vi "Update Analysis DVR U16.vi"(8 "error in (no error)":errorcluster, 9 "images":refnum<data-value>[](array[refnum]), 10 "Analysis Image":dbl[][](array[numeric]), 11 "Analysis Graph in":refnum<class "Analysis Graph.lvclass">) -> (0 "error out":errorcluster, 1 "pixel signal roied":u16[](array[numeric]), 2 "Cursor.Cursor Position":T1, 3 "Analysis Graph out":refnum<class "Analysis Graph.lvclass">)   [LabVIEW 2023, in "Analysis Graph.lvclass"]
uses:
  Analysis Graph.lvclass
  Series Graph/Series Graph.lvclass
  Detail Graph/Detail Graph.lvclass
  <vilib>/Utility/miscctls.llb/LVPointDoubleTypeDef.ctl
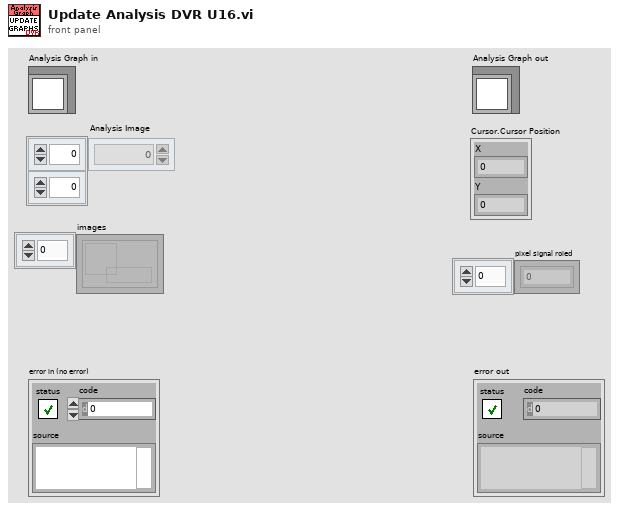
[diagram p1: front panel]
types:
  T1 = typedef "LVPointDoubleTypeDef.ctl" = cluster{"X":dbl, "Y":dbl}
  T2 = cluster{"ROI X":cluster{"Index":u32, "Length":u32}, "ROI Y":cluster{"Index":u32, "Length":u32}, "ROI Z":cluster{"Index":u32, "Length":u32}}
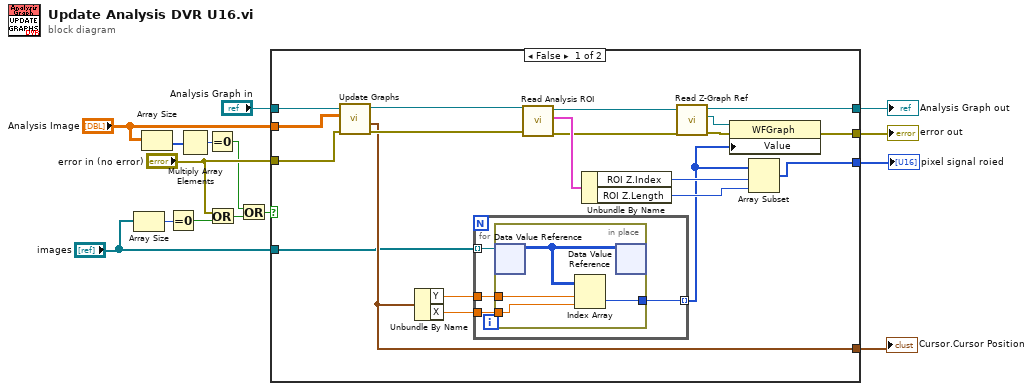
[diagram p0: block diagram]
diagram:
  n1 = Array Size(array="images") -> (size(s)=w8:i32)
  n2 = Array Size(array="Analysis Image") -> (size(s)=w4:i32[])
  n3 = Equal To 0?(x=w8) -> (x = 0?=w12:bool)
  n4 = Multiply Array Elements(1:w4) -> (0:w3:i32)
  n5 = Equal To 0?(x=w3) -> (x = 0?=w1:bool)
  n6 = Or(x="error in (no error)", y=w12) -> (x .or. y?=w11:bool)
  n7 = Or(x=w1, y=w11) -> (x .or. y?=w2:bool)
  n8 = case shown="False" w2 {
    tunnel: [w31 w44] -> w15
    tunnel: [w35 w45] -> w13
    tunnel: "Analysis Graph in" -> [w27 w45]
    tunnel: "error in (no error)" -> [w26 w44]
    tunnel: "Analysis Image" -> [w32 _]
    tunnel: "images" -> [w18 _]
    tunnel: [w19 _] -> w9
    tunnel: [w16 _] -> w6
    frame False {
      n9 = call "Update Graphs.vi"("error in (no error)"=w26, "image"=w32, "Detail Graph in"=w27) -> ("error out"=w29:errorcluster, "Cursor.Cursor Position"=w19:T1, "Detail Graph out"=w23:refnum<class "Analysis Graph.lvclass">)  [unwired: 6 in]
      n10 = Unbundle By Name(w19) -> ("Y"=w21:dbl, "X"=w20:dbl)
      n11 = for {
        tunnel: w18 -> [w39] mode=indexing
        tunnel: w21 -> [w38]
        tunnel: w20 -> [w37]
        tunnel: [w36] -> w17 mode=indexing
        n12 = in-place {
          in-place-border: w38 -> [w43]
          in-place-border: w37 -> [w42]
          in-place-border: [w41] -> w36
          n13 = in-place-dvr #1(w39) -> (w40:u16[][])  [unwired: 1 out]
          n14 = Index Array(array=w40, index (row)=w43, index (col)=w42) -> (element=w41:u16)
          n15 = in-place-dvr #1(w40) -> ()  [unwired: 2 out]
        }
      }
      n16 = call "Read Analysis ROI.vi"("error in (no error)"=w29, "Analysis Graph in"=w23) -> ("error out"=w28:errorcluster, "ROI XYZ"=w30:T2, "Analysis Graph out"=w22:refnum<class "Analysis Graph.lvclass">)  [unwired: 7 in]
      n17 = Unbundle By Name(w30) -> ("ROI Z.Index"=w25:u32, "ROI Z.Length"=w24:u32)
      n18 = call "Read Z-Graph Ref.vi"("error in (no error)"=w28, "Series Graph in"=w22) -> ("error out"=w33:errorcluster, "Z-Graph Ref"=w34:refnum<vi>, "Series Graph out"=w35:refnum<class "Analysis Graph.lvclass">)  [unwired: 7 in]
      n19 = property class="WFGraph"(reference=w34, error in=w33, "Value"=w17) -> (error out=w31:errorcluster)  [unwired: 1 out]
      n20 = Array Subset(array=w17, index=w25, length=w24) -> (w16:u16[])
    }
    frame True {
    }
  }
  "error out" <- w15
  "Analysis Graph out" <- w13
  "Cursor.Cursor Position" <- w9
  "pixel signal roied" <- w6
